vi "ClawNetwork.vi"(8 "error in (no error)":errorcluster) -> (0 "error out":errorcluster)   [LabVIEW 2020]
doc: "Claw network\n\nInputs:\n -- Error in -- Error cluster -- propagated error input\n\nOutputs:\n -- Error out -- Error cluster -- progated error output"
uses:
  ClawGlobal.vi
  <vilib>/Rock Robotics/Network Tables/NT Write Number.vi
  <vilib>/Rock Robotics/Network Tables/NT Write Boolean.vi
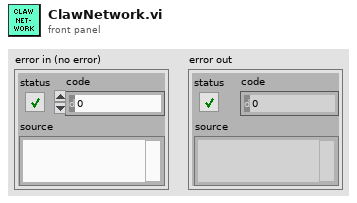
[diagram p1: front panel]
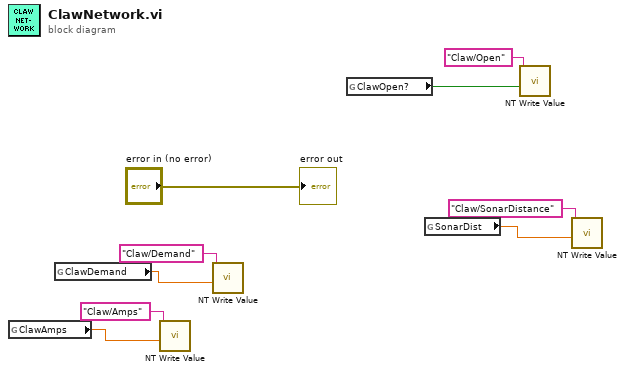
[diagram p0: block diagram]
diagram:
  n1 = global read "ClawGlobal.vi" "ClawAmps"() -> (w2:dbl)
  n2 = global read "ClawGlobal.vi" "ClawDemand"() -> (w6:dbl)
  n3 = call-poly <vilib>:"NT Write Value.vi"("value"=w2, "name"="Claw/Amps") -> ()  [unwired: 9 in, 1 out]
  n4 = call-poly <vilib>:"NT Write Value.vi"("value"=w6, "name"="Claw/Demand") -> ()  [unwired: 9 in, 1 out]
  n5 = global read "ClawGlobal.vi" "ClawOpen?"() -> (w8:bool)
  n6 = global read "ClawGlobal.vi" "SonarDist"() -> (w4:dbl)
  n7 = call-poly <vilib>:"NT Write Value.vi"("value"=w8, "name"="Claw/Open") -> ()  [unwired: 9 in, 1 out]
  n8 = call-poly <vilib>:"NT Write Value.vi"("value"=w4, "name"="Claw/SonarDistance") -> ()  [unwired: 9 in, 1 out]
  "error out" <- "error in (no error)"
